vi "VelMove.vi"(8 "error in (no error)":errorcluster, 11 "Axis in":refnum<class "Axis.lvclass">) -> (0 "error out":errorcluster, 3 "Axis out":refnum<class "Axis.lvclass">)   [LabVIEW 2020, in "Axis.lvclass"]
uses:
  Axis.lvclass
  Axis.lvclass/Axis.ctl
  C:/Users/Jonathan/Documents/Clearpath SDK/CSharp Examples/CLRWrapper/x64/Debug/CLRWrapper.dll
  CSharp Examples/CLRWrapper/x64/Debug/CLRWrapper.dll
panel:
  in  "targetVel":dbl
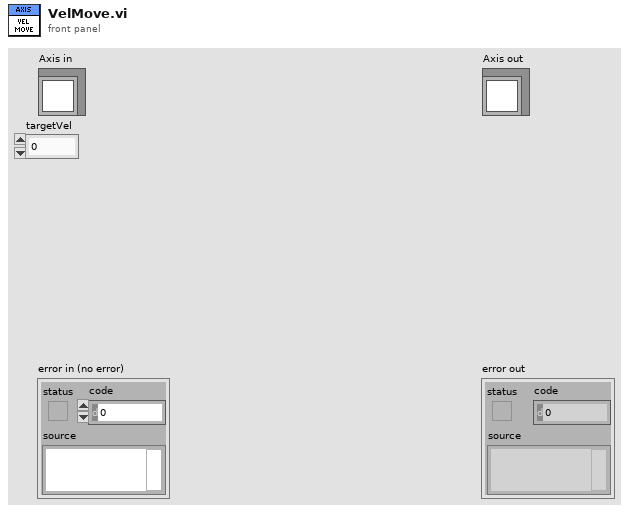
[diagram p1: front panel]
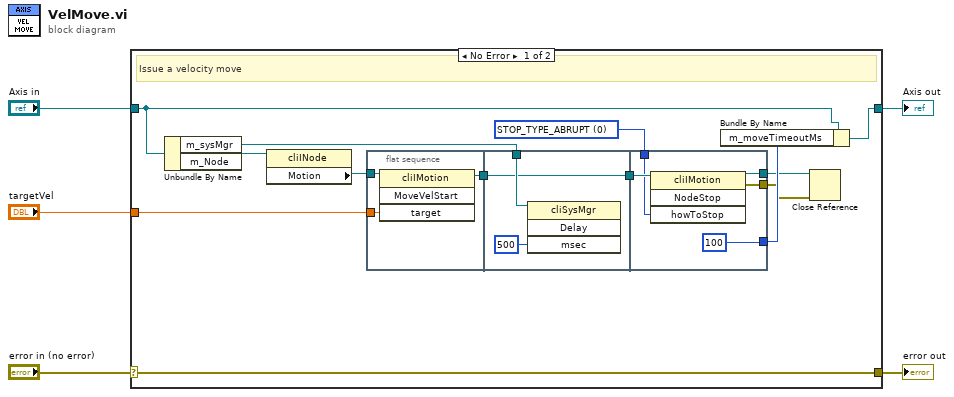
[diagram p0: block diagram]
diagram:
  n1 = case shown="No Error" "error in (no error)" {
    selector: "error in (no error)" -> [w18 w31]
    tunnel: [w18 w31] -> w4
    tunnel: [w10 w30] -> w2
    tunnel: "Axis in" -> [w9 w30]
    tunnel: "targetVel" -> [w15 _]
    frame No Error {
      w11 = 0 items=["STOP_TYPE_ABRUPT"=0, "STOP_TYPE_RAMP"=1, "STOP_TYPE_IGNORE"=3, "STOP_TYPE_RAMP_AT_DECEL"=4, "STOP_TYPE_ESTOP_ABRUPT"=16, "STOP_TYPE_ESTOP_RAMP"=17, "STOP_TYPE_ESTOP_RAMP_AT_DECEL"=20, "STOP_TYPE_CLR_ESTOP"=24, "STOP_TYPE_CLR_CTRLD"=40, "STOP_TYPE_DISABLE_ABRUPT, STOP_TYPE_DISABLE_RAMP_AT_DECEL, STOP_TYPE_DISABLE_RAMP"=128, "STOP_TYPE_CLR_DISABLE"=136, "STOP_TYPE_ESTOP_DISABLE_RAMP"=145, "STOP_TYPE_CLR_ALL"=248] ("howToStop")
      # "Issue a velocity move"
      n2 = Unbundle By Name(w9) -> ("m_sysMgr"=w14:refnum<k24>, "m_Node"=w17:refnum<k24>)
      n3 = property class="cliINode"(reference=w17) -> ("Motion"=w16:refnum<k24>)  [unwired: 1 in, 2 out]
      n4 = flat-sequence {
        tunnel: w16 -> [w21]
        tunnel: w15 -> [w20]
        tunnel: [w19] -> w13
        tunnel: w14 -> [w24]
        tunnel: w13 -> [w22]
        tunnel: [w22] -> w12
        tunnel: w12 -> [w29]
        tunnel: w11 -> [w28]
        tunnel: [100 ("m_moveTimeoutMs")] -> w8
        tunnel: [w26] -> w7
        tunnel: [w25] -> w6
        frame #0 {
          n5 = invoke class="cliIMotion" method="MoveVelStart"(reference=w21, "target"=w20) -> (reference out=w19:refnum<k24>)  [unwired: 2 in, 3 out]
        }
        frame #1 {
          n6 = invoke class="cliSysMgr" method="Delay"(reference=w24, "msec"=u32 500) -> ()  [unwired: 2 in, 4 out]
        }
        frame #2 {
          n7 = invoke class="cliIMotion" method="NodeStop"(reference=w29, "howToStop"=w28) -> (reference out=w26:refnum<k24>, error out=w25:errorcluster)  [unwired: 2 in, 2 out]
        }
      }
      n8 = Bundle By Name(cluster=w9, "m_moveTimeoutMs"=w8) -> (w10:refnum<class "Axis.lvclass">)
      n9 = Close Reference(reference=w7, error in (no error)=w6) -> ()  [unwired: 1 out]
    }
    frame Error {
    }
  }
  "error out" <- w4
  "Axis out" <- w2
